vi "Deinitialize Sync Stuff.vi"(8 "error in (no error)":errorcluster, 11 "IP Connection in":refnum<class "IP Connection.lvclass">) -> (0 "error out":errorcluster, 3 "IP Connection out":refnum<class "IP Connection.lvclass">)   [LabVIEW 2011, in "Tinkerforge.lvlib" / "IP Connection.lvclass"]
doc: "This VI deinitializes the synchronization objects of the IP connection object."
uses:
  IP Connection.lvclass
  IP Connection.lvclass/IP Connection.ctl
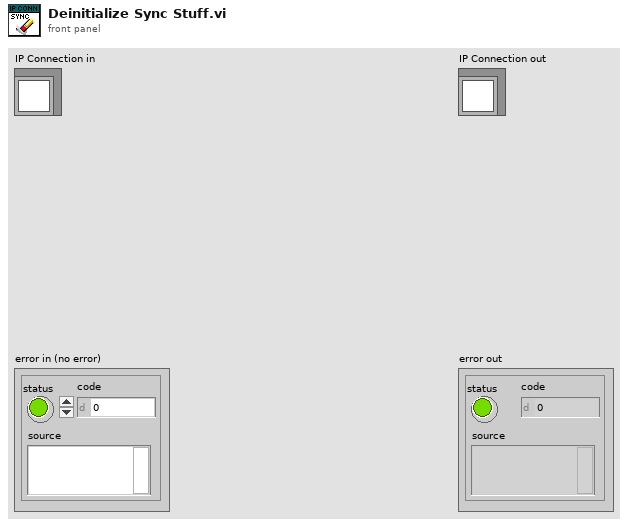
[diagram p1: front panel]
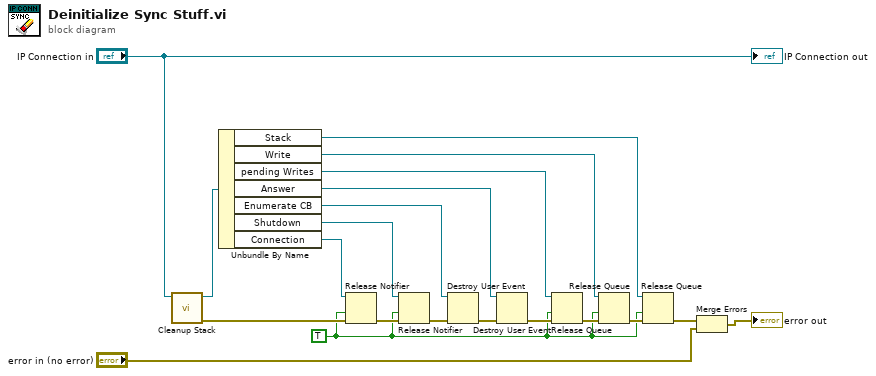
[diagram p0: block diagram]
diagram:
  w2 = TRUE ("force destroy? (F)")
  n1 = call "Cleanup Stack.vi"("IP Connection in"="IP Connection in") -> ("error out"=w3:errorcluster, "IP Connection out"=w5:refnum<class "IP Connection.lvclass">)  [unwired: 9 in]
  n2 = Unbundle By Name(w5) -> ("Stack"=w9:refnum<queue>, "Write"=w19:refnum<queue>, "pending Writes"=w20:refnum<queue>, "Answer"=w16:refnum<user-event>, "Enumerate CB"=w14:refnum<user-event>, "Shutdown"=w10:refnum<notifier>, "Connection"=w1:refnum<notifier>)
  n3 = Release Notifier(notifier=w1, force destroy? (F)=w2, error in (no error)=w3) -> (error out=w4:errorcluster)  [unwired: 2 out]
  n4 = Release Notifier(notifier=w10, force destroy? (F)=w2, error in (no error)=w4) -> (error out=w11:errorcluster)  [unwired: 2 out]
  n5 = Destroy User Event(user event=w14, error in=w11) -> (error out=w15:errorcluster)
  n6 = Destroy User Event(user event=w16, error in=w15) -> (error out=w17:errorcluster)
  n7 = Release Queue(queue=w20, force destroy? (F)=w2, error in (no error)=w17) -> (error out=w18:errorcluster)  [unwired: 2 out]
  n8 = Release Queue(queue=w19, force destroy? (F)=w2, error in (no error)=w18) -> (error out=w8:errorcluster)  [unwired: 2 out]
  n9 = Release Queue(queue=w9, force destroy? (F)=w2, error in (no error)=w8) -> (error out=w7:errorcluster)  [unwired: 2 out]
  n10 = Merge Errors(w7, "error in (no error)") -> (→"error out":errorcluster)
  "IP Connection out" <- "IP Connection in"
